vi "wrap_DigitalOut.vi"(3 "State":bool, 4 "Component ID":u16(ring) items=["left_itb_light_inner", "right_itb_light_inner", "torso_left_itb_light_inner", "torso_right_itb_light_inner", "left_itb_light_outer", "right_itb_light_outer", "torso_left_itb_light_outer", "torso_right_itb_light_outer"], 5 "msg in":string) -> (2 "msg out":string)   [LabVIEW 2012]
doc: "Flattens a wrap digital out into a message"
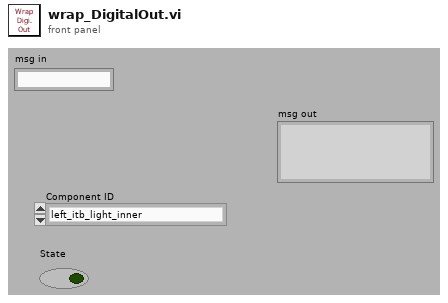
[diagram p1: front panel]
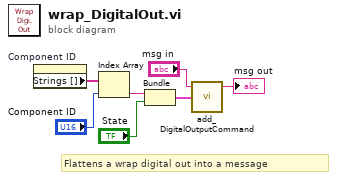
[diagram p0: block diagram]
diagram:
  # "Flattens a wrap digital out into a message"
  n1 = property on="Component ID" class="Ring (strict)"() -> ("Strings []"=w2:string[])  [unwired: 2 in, 2 out]
  n2 = Index Array(array=w2, index="Component ID") -> (element=w5:string)
  n3 = Bundle(w5, "State"="State") -> (w7:cluster{string, "State":bool})  [unwired: 1 in]
  n4 = call <userlib>:"add_DigitalOutputCommand.vi"("Digital Output Command"=w7, "msg in"="msg in") -> ("msg out"=→"msg out":string)  [unwired: 3 in]
